vi "FRCts20_Backend_GenIssueTeamList.vi"(8 "error in (no error)":errorcluster, 11 "Competitions":T1) -> (0 "error out":errorcluster, 2 "IssueTeamList":string, 3 "Competitions Oot":T1)   [LabVIEW 2013, in "FRCts20_Backend_Engine_Deprecated.lvlib"]
uses:
  FRCts20_Backend_Engine_Deprecated.lvlib
  FRCts20_Backend_TeamLocation.ctl
  FRCts20_Backend_Controls.lvlib
  FRCts20_Backend_IssueDfn.ctl
  FRCts20_Backend_TeamDfn.ctl
  FRCts20_Backend_TeamDataDfn.ctl
  FRCts20_Backend_IssueTeamList.ctl
  FRCts20_Backend_Team_Info.ctl
  FRCts20_Backend_Note.ctl
  FRCts20_Backend_Note_list.ctl
  FRCts20_Backend_request_info.ctl
  FRCts20_Backend_Competition_Info.ctl
  FRCts20_Backend_Division_Info.ctl
  FRCts20_Backend_Division.ctl
  FRCts20_Backend_Division_List.ctl
  FRCts20_Backend_Competition.ctl
  FRCts20_Backend_Competition_List.ctl
panel:
  in  "IssueTeamList_Ref":T10
  in  "Team_Ref":T16
  in  "IssueTeamList_Init":T10
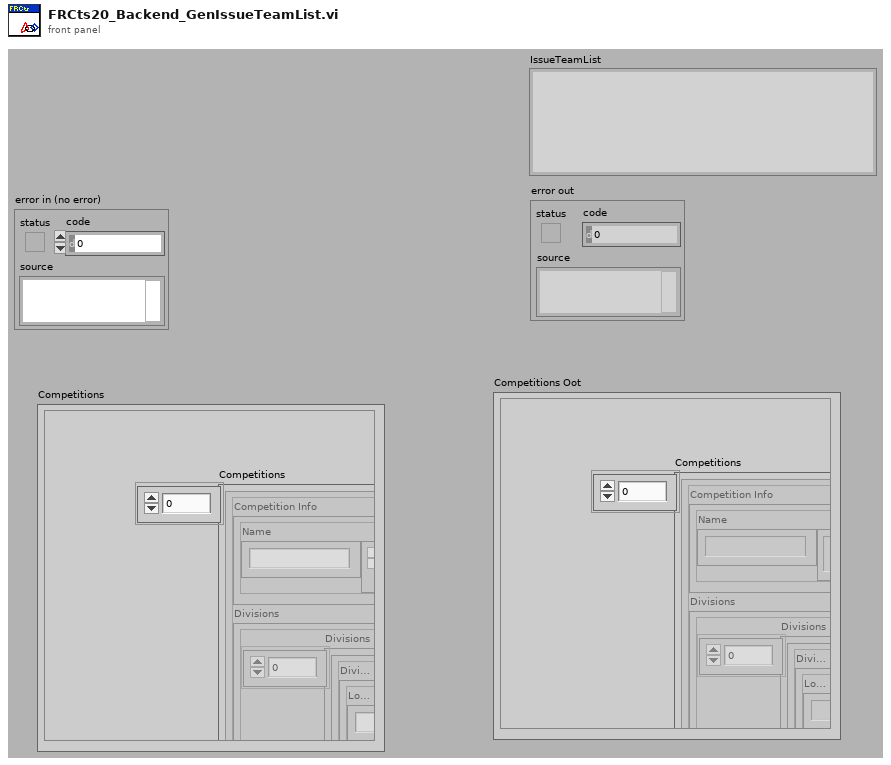
[diagram p1: front panel]
types:
  T1 = typedef "FRCts20_Backend_Controls.lvlib/FRCts20_Backend_Competition_List.ctl" = cluster{"Competitions":T2[]}
  T2 = typedef "FRCts20_Backend_Controls.lvlib/FRCts20_Backend_Competition.ctl" = cluster{"Competition Info":T3, "Divisions":T4}
  T3 = typedef "FRCts20_Backend_Controls.lvlib/FRCts20_Backend_Competition_Info.ctl" = cluster{"Name":string, "Start Date":timestamp, "Duration":u8}
  T4 = typedef "FRCts20_Backend_Controls.lvlib/FRCts20_Backend_Division_List.ctl" = cluster{"Divisions":T5[]}
  T5 = typedef "FRCts20_Backend_Controls.lvlib/FRCts20_Backend_Division.ctl" = cluster{"Division Info":T6, "TeamData":T7}
  T6 = typedef "FRCts20_Backend_Controls.lvlib/FRCts20_Backend_Division_Info.ctl" = cluster{"Location":string}
  T7 = typedef "FRCts20_Backend_Controls.lvlib/FRCts20_Backend_TeamDataDfn.ctl" = cluster{"Team":T8[]}
  T8 = typedef "FRCts20_Backend_Controls.lvlib/FRCts20_Backend_TeamDfn.ctl" = cluster{"Team Info":T9, "IssueList":T10}
  T9 = typedef "FRCts20_Backend_Controls.lvlib/FRCts20_Backend_Team_Info.ctl" = cluster{"TeamNumber":u16, "SWType":string}
  T10 = typedef "FRCts20_Backend_Controls.lvlib/FRCts20_Backend_IssueTeamList.ctl" = cluster{"Issues":T11[]}
  T11 = typedef "FRCts20_Backend_Controls.lvlib/FRCts20_Backend_IssueDfn.ctl" = cluster{"Notes":T12, "Info":T14}
  T12 = typedef "FRCts20_Backend_Controls.lvlib/FRCts20_Backend_Note_list.ctl" = cluster{"Notes":T13[]}
  T13 = typedef "FRCts20_Backend_Controls.lvlib/FRCts20_Backend_Note.ctl" = cluster{"Time Entered":timestamp, "Author":string, "Text":string}
  T14 = typedef "FRCts20_Backend_Controls.lvlib/FRCts20_Backend_request_info.ctl" = cluster{"Status":enum16{"Open", "In Work", "Closed"}, "Open Date":timestamp, "Description":string, "Last Update":timestamp, "Closed Date":timestamp, "Solution Index":i32}
  T15 = typedef "FRCts20_Backend_Controls.lvlib/FRCts20_Backend_TeamLocation.ctl" = string
  T16 = cluster{"SetTime":timestamp, "TeamNumber":u16, "Location":T15, "Description":string}
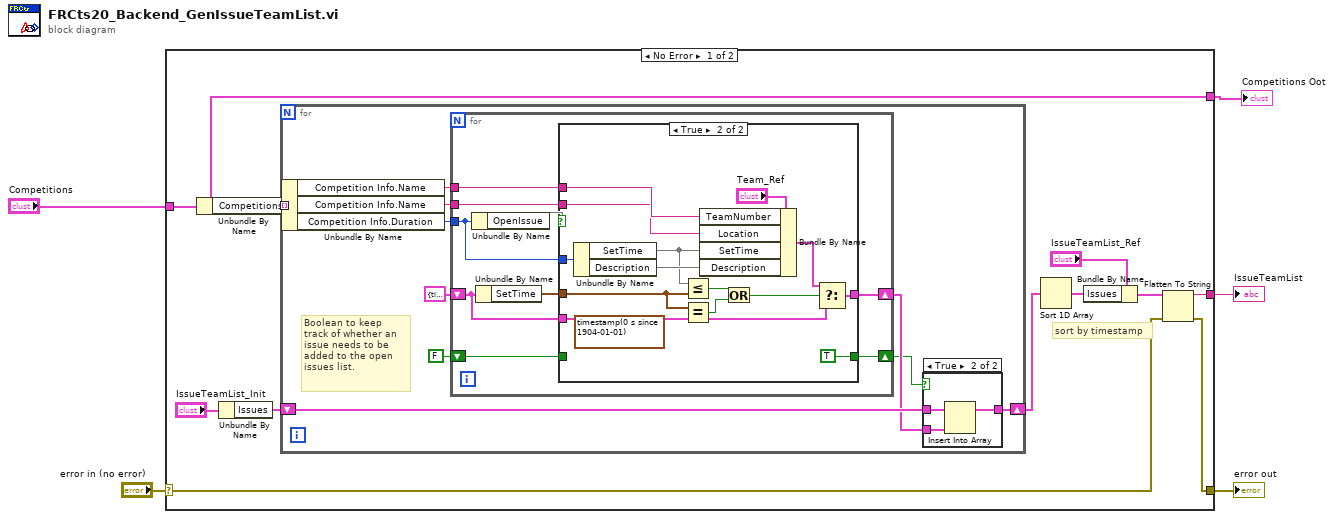
[diagram p0: block diagram]
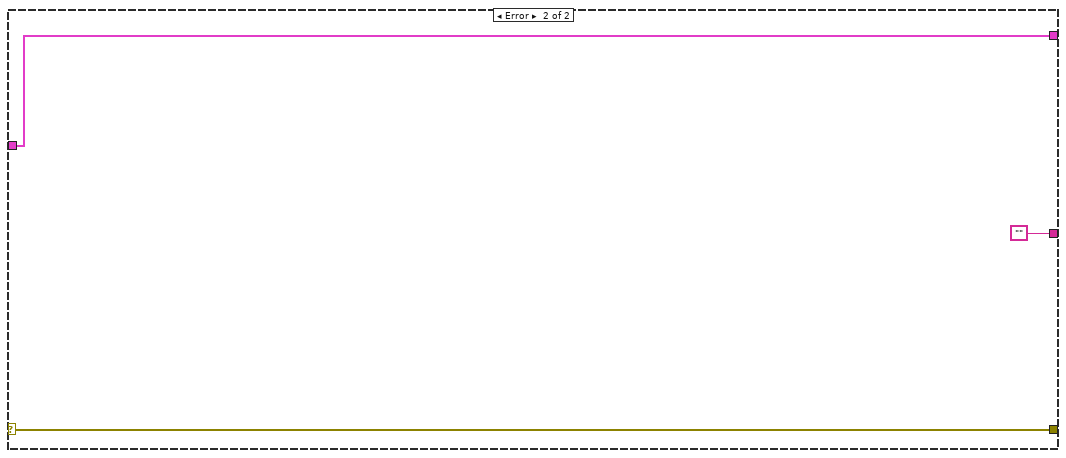
[diagram p4: hidden frame]
diagram:
  n1 = case shown="No Error" "error in (no error)" {
    selector: "error in (no error)" -> [w7 w59]
    tunnel: [w6 w59] -> w4
    tunnel: "Competitions" -> [w10 w57]
    tunnel: [w10 w57] -> w1
    tunnel: [w8 ""] -> w3
    frame No Error {
      # "sort by timestamp"
      n2 = Unbundle By Name(w10) -> ("Competitions"=w16:T2[])
      n3 = Unbundle By Name("IssueTeamList_Init") -> ("Issues"=w14:T11[])
      n4 = for {
        tunnel: w16 -> [w26] mode=indexing
        shift-right: [w21] -> w13
        shift-left: w14 -> [w22]
        # "Boolean to keep \ntrack of whether an \nissue needs to be \nadded to the open \nissues list."
        n5 = Unbundle By Name(w26) -> ("Competition Info.Name"=w25:string, "Competition Info.Name"=w24:string, "Competition Info.Duration"=w19:u8)
        n6 = for {
          tunnel: w19 -> [w38]
          tunnel: w25 -> [w37]
          tunnel: w24 -> [w36]
          shift-right: [w33] -> w20
          shift-left: T16 {"SetTime"=timestamp(0 s since 1904-01-01), "TeamNumber"=0, "Location"="", "Description"=""} ("Team_Ref 2") -> [w34]
          shift-right: [w31] -> w17
          shift-left: FALSE -> [w32]
          n7 = Unbundle By Name(w38) -> ("OpenIssue"=w39)
          n8 = Unbundle By Name(w34) -> ("SetTime"=w35:timestamp)
          n9 = case shown="True" w39 {
            tunnel: w38 -> [_ w56]
            tunnel: w37 -> [_ w53]
            tunnel: w36 -> [_ w52]
            tunnel: w35 -> [_ w45]
            tunnel: w34 -> [w41 w51]
            tunnel: [w41 w50] -> w33
            tunnel: w32 -> [w40 _]
            tunnel: [w40 TRUE] -> w31
            frame False {
            }
            frame True {
              n10 = Unbundle By Name(w56) -> ("SetTime"=w49, "Description"=w55)
              n11 = Less Or Equal?(x=w49, y=w45) -> (x <= y?=w47:bool)
              n12 = Equal?(x=w45, y=timestamp(0 s since 1904-01-01)) -> (x = y?=w44:bool)
              n13 = Bundle By Name(cluster="Team_Ref", "TeamNumber"=w53, "Location"=w52, "SetTime"=w49, "Description"=w55) -> (w48:T16)
              n14 = Or(x=w47, y=w44) -> (x .or. y?=w46:bool)
              n15 = Select(t=w48, s=w46, f=w51) -> (s? t:f=w50:T16)
            }
          }
        }
        n16 = case shown="True" w17 {
          tunnel: w22 -> [w27 w30]
          tunnel: [w27 w29] -> w21
          tunnel: w20 -> [_ w28]
          frame False {
          }
          frame True {
            n17 = Insert Into Array(array=w30, new element=w28) -> (w29:T11[])  [unwired: 1 in]
          }
        }
      }
      n18 = Sort 1D Array(array=w13) -> (sorted array=w11:T11[])
      n19 = Bundle By Name(cluster="IssueTeamList_Ref", "Issues"=w11) -> (w9:T10)
      n20 = Flatten To String(anything=w9, error in (no error)=w7) -> (data string=w8:string, error out=w6:errorcluster)  [unwired: 2 in, 1 out]
    }
    frame Error {
    }
  }
  "error out" <- w4
  "IssueTeamList" <- w3
  "Competitions Oot" <- w1
